vi "Create_Event_ToMessageHandler.vi"(8 "Error in":errorcluster, 11 "EVE reference in":refnum<data-value>) -> (0 "Error out":errorcluster, 3 "EVE reference out":refnum<data-value>)   [LabVIEW 2013, in "EVE.lvclass"]
uses:
  EVE.lvclass
  030 - EVENTS/EnumFgvEventCommand.ctl
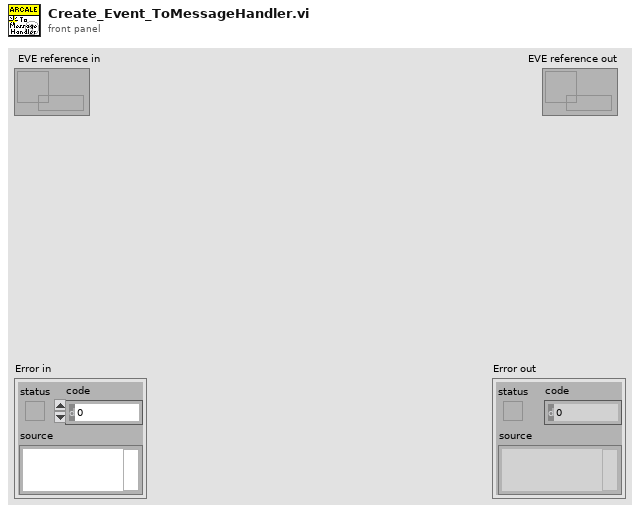
[diagram p1: front panel]
types:
  T1 = typedef "EnumFgvEventCommand.ctl" = enum16{"Setup", "Cleanup", "Get"}
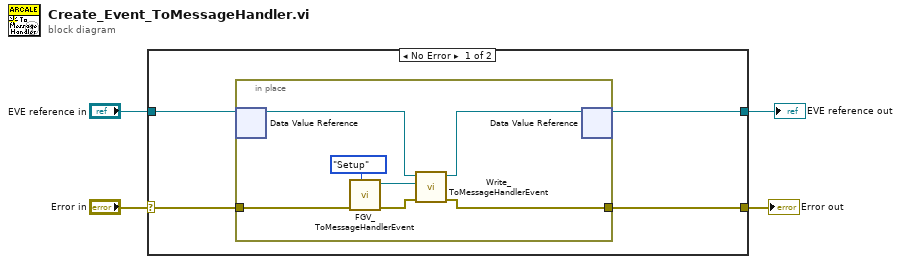
[diagram p0: block diagram]
diagram:
  n1 = case shown="No Error" "Error in" {
    selector: "Error in" -> [w8 w17]
    tunnel: [w7 w17] -> w3
    tunnel: "EVE reference in" -> [w6 w16]
    tunnel: [w5 w16] -> w1
    frame No Error {
      n2 = in-place {
        in-place-border: w8 -> [w13]
        in-place-border: [w12] -> w7
        n3 = in-place-dvr #1(w6) -> (w11:refnum<class "EVE.lvclass">)  [unwired: 1 out]
        n4 = call "FGV_ToMessageHandlerEvent.vi"("Command"=EnumFgvEventCommand."Setup", "error in (no error)"=w13) -> ("error out"=w14:errorcluster, "To message handler event"=w9:refnum<user-event>)  [unwired: 8 in]
        n5 = call-dynamic "Write_ToMessageHandlerEvent.vi"("error in (no error)"=w14, "To message handler event"=w9, "EVE in"=w11) -> ("error out"=w12:errorcluster, "EVE out"=w10:refnum<class "EVE.lvclass">)  [unwired: 7 in]
        n6 = in-place-dvr #1(w10) -> (w5:refnum<data-value>)  [unwired: 1 out]
      }
    }
    frame Error {
    }
  }
  "Error out" <- w3
  "EVE reference out" <- w1
